vi "Bundle Script_Named (Un)Bundler Rearrange.vi"(8 "error in":errorcluster, 10 "Displayed Items":string[](array[string]), 11 "Affected Items":T1) -> (0 "error out":errorcluster, 2 "Objects":refnum<vi>[](array[refnum]))   [LabVIEW 2023]
doc: "Tag tree tags as nput, as these contain the original indices, which are used for reordering the wires and labels of the bundle or unbundle by name structures"
uses:
  top/BundleMagic.ctl
panel:
  out "Array":cluster{"Array":bool[]}[](array[cluster])
  out "Bundle Type":T2(ring)
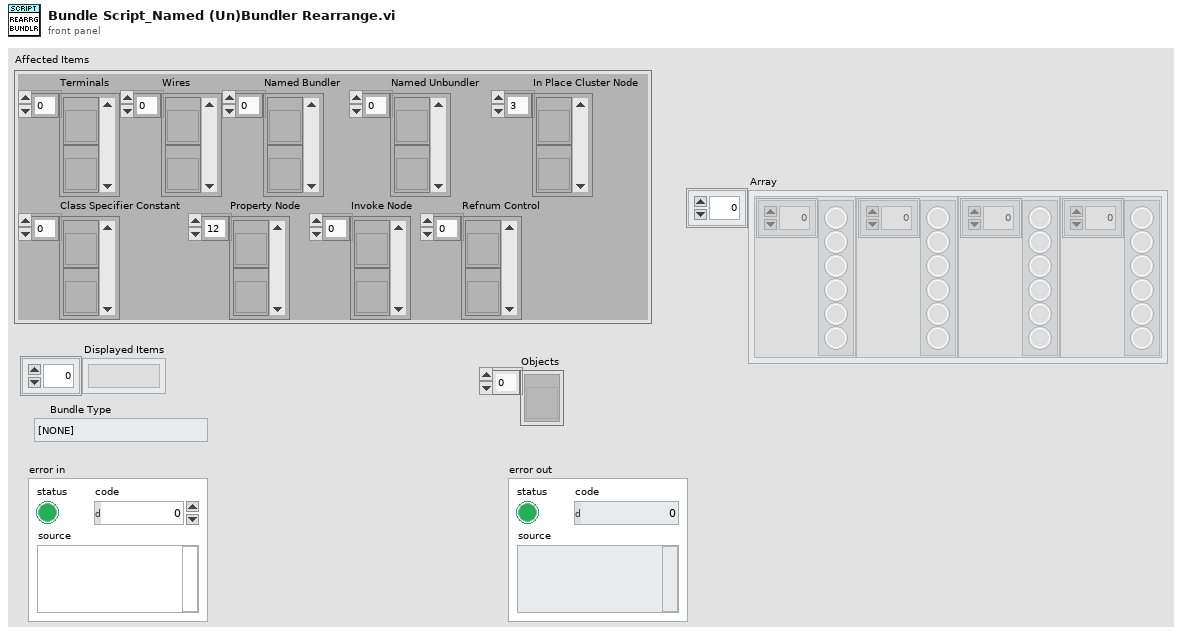
[diagram p1: front panel]
types:
  T1 = typedef "BundleMagic.ctl" = cluster{"Terminals":refnum<vi>[], "Wires":refnum<vi>[], "Named Bundler":refnum<vi>[], "Named Unbundler":refnum<vi>[], "In Place Cluster Node":refnum<vi>[], "Class Specifier Constant":refnum<vi>[], "Property Node":refnum<vi>[], "Invoke Node":refnum<vi>[], "Refnum Control":refnum<vi>[]}
  T2 = enum16{"[NONE]", "Unbundle", "Bundle", "Insert Before", "Insert After", "Remove Elements", "Rearrange Elements"}
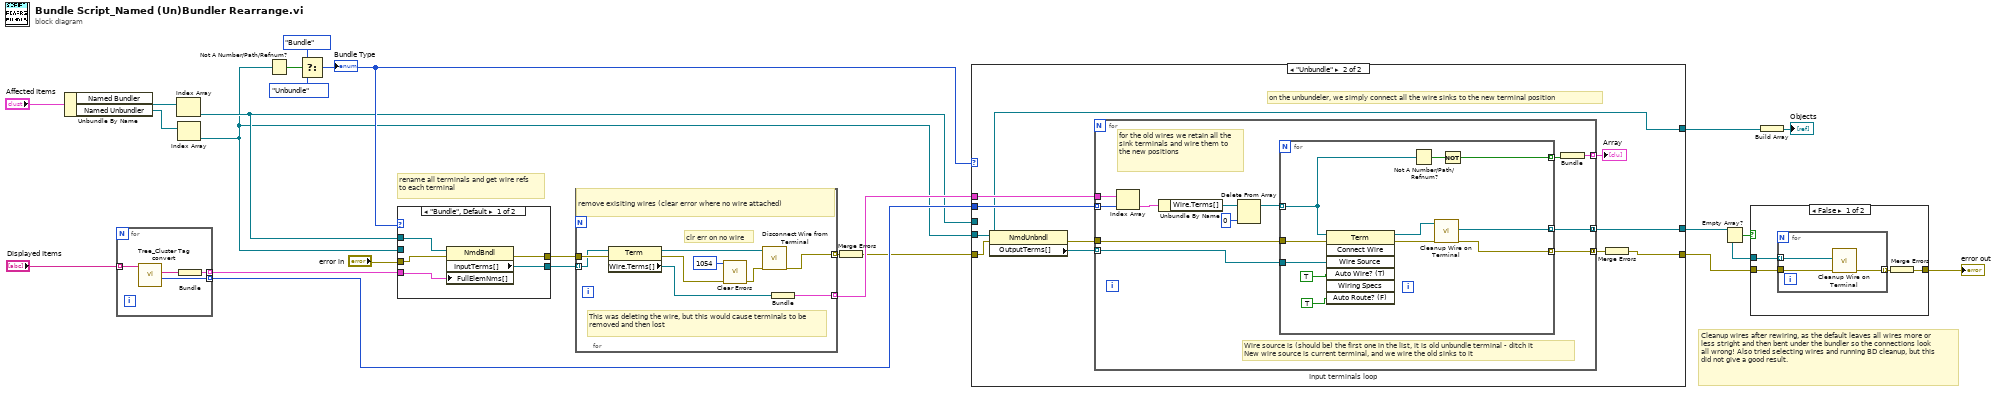
[diagram p0: block diagram]
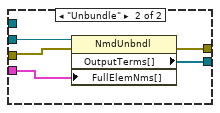
[diagram p2: hidden frame]
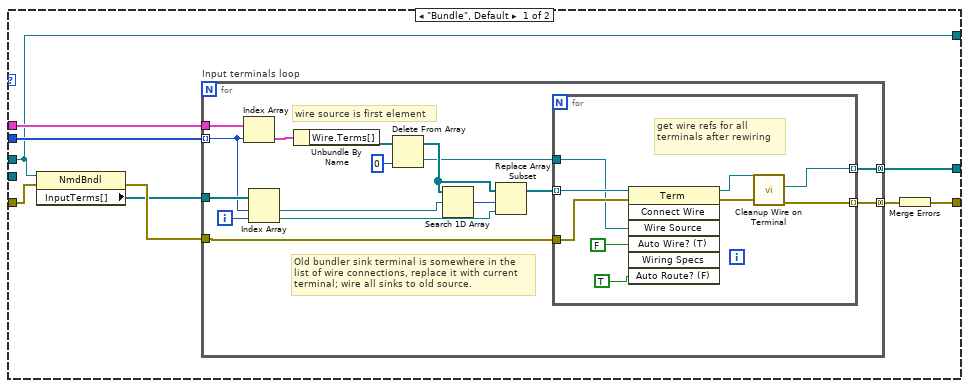
[diagram p3: hidden frame]
diagram:
  # "Cleanup wires after rewiring, as the default leaves all wires more or less stright and then bent under the bundler so the connections look all wrong! Also tried selecting wires and running BD cleanup, but this did not give a good result."
  # "rename all terminals and get wire refs to each terminal"
  n1 = Unbundle By Name("Affected Items") -> ("Named Bundler"=w14:refnum<vi>[], "Named Unbundler"=w12:refnum<vi>[])
  n2 = for {
    tunnel: "Displayed Items" -> [w28] mode=indexing
    tunnel: [w25] -> w17 mode=indexing
    tunnel: [w26] -> w19 mode=indexing
    n3 = call "Tree_Cluster Tag convert.vi"("Tag"=w28) -> ("Index"=w26:u32, "Tree Nest"=w27:string[])  [unwired: 5 in, 4 out]
    n4 = Bundle("Tree Nest"=w27) -> (w25:cluster{"Tree Nest":string[]})  [unwired: 1 in]
  }
  n5 = Index Array(array=w14) -> (element=w11:refnum<vi>)  [unwired: 1 in]
  n6 = Index Array(array=w12) -> (element=w9:refnum<vi>)  [unwired: 1 in]
  n7 = Not A Number/Path/Refnum?(number/path/refnum=w9) -> (NaN/Path/Refnum?=w10:bool)
  n8 = Select(t=T2."Bundle" ("Action"), s=w10, f=T2."Unbundle" ("Action")) -> (s? t:f=w16:T2)
  "Bundle Type" <- w16
  n9 = case shown="\"Bundle\", Default" w16 {
    tunnel: [w30 w38] -> w21
    tunnel: [w31 w37] -> w24
    tunnel: w11 -> [w33 _]
    tunnel: w17 -> [w32 w35]
    tunnel: w9 -> [_ w36]
    tunnel: "error in" -> [w29 w34]
    frame "Bundle", Default {
      n10 = property class="NmdBndl"(reference=w33, error in=w29, "FullElemNms[]"=w32) -> (error out=w31:errorcluster, "InputTerms[]"=w30:refnum<vi>[])  [unwired: 1 out]
    }
    frame "Unbundle" {
      n11 = property class="NmdUnbndl"(reference=w36, error in=w34, "FullElemNms[]"=w35) -> (error out=w37:errorcluster, "OutputTerms[]"=w38:refnum<vi>[])  [unwired: 1 out]
    }
  }
  n12 = for {
    tunnel: w21 -> [w46] mode=indexing
    tunnel: [w44] -> w20 mode=indexing
    tunnel: w24 -> [w47]
    tunnel: [w41] -> w18 mode=indexing
    # "This was deleting the wire, but this would cause terminals to be removed and then lost"
    # "clr err on no wire"
    # "remove exisiting wires (clear error where no wire attached)"
    n13 = property class="Term"(reference=w46, error in=w47) -> (reference out=w43:refnum<vi>, error out=w42:errorcluster, "Wire.Terms[]"=w45:refnum<vi>[])
    n14 = call <vilib>:"Clear Errors.vi"("error in (no error)"=w42, "specific error code to clear (0: all)"=1054) -> ("error out"=w40:errorcluster)  [unwired: 4 in, 1 out]
    n15 = call "Disconnect Wire from Terminal.vi"("error in"=w40, "Terminal in"=w43) -> ("error out"=w41:errorcluster)  [unwired: 5 in, 4 out]
    n16 = Bundle("Wire.Terms[]"=w45) -> (w44:cluster{"Wire.Terms[]":refnum<vi>[]})  [unwired: 1 in]
  }
  n17 = Merge Errors(w18) -> (w1:errorcluster)
  n18 = case shown="\"Unbundle\"" w16 {
    tunnel: w1 -> [w53 w88]
    tunnel: w20 -> [w55 w90]
    tunnel: w11 -> [w49 _]
    tunnel: w9 -> [_ w83]
    tunnel: w19 -> [w52 w87]
    tunnel: [w51 w85] -> w3
    tunnel: [w48 w82] -> w8
    tunnel: [w49 w83] -> w5
    frame "Bundle", Default {
      n19 = property class="NmdBndl"(reference=w49, error in=w53) -> (error out=w56:errorcluster, "InputTerms[]"=w54:refnum<vi>[])  [unwired: 1 out]
      n20 = for "Input terminals loop" {
        tunnel: w55 -> [w71]
        tunnel: w52 -> [w68] mode=indexing
        tunnel: w54 -> [w69]
        tunnel: w56 -> [w72]
        tunnel: [w58] -> w51 mode=concatenating
        tunnel: [w57] -> w50 mode=concatenating
        i -> [w67]
        # "wire source is first element"
        # "Old bundler sink terminal is somewhere in the list of wire connections, replace it with current terminal; wire all sinks to old source."
        n21 = Index Array(array=w71, index=w68) -> (element=w70:cluster{"Wire.Terms[]":refnum<vi>[]})
        n22 = Index Array(array=w69, index #1=w68, index #2=w67) -> (element #1=w65:refnum<vi>, element #2=w63:refnum<vi>)
        n23 = Unbundle By Name(w70) -> ("Wire.Terms[]"=w66:refnum<vi>[])
        n24 = Delete From Array(array=w66, index=0) -> (deleted portion=w59:refnum<vi>, array with subset deleted=w61:refnum<vi>[])  [unwired: 1 in]
        n25 = Search 1D Array(1D array=w61, element=w65) -> (index of element=w64:i32)  [unwired: 1 in]
        n26 = Replace Array Subset(array=w61, new element=w63, index=w64) -> (w62:refnum<vi>[])
        n27 = for {
          tunnel: w72 -> [w81]
          tunnel: w62 -> [w80] mode=indexing
          tunnel: w59 -> [w78]
          tunnel: [w74] -> w58 mode=indexing
          tunnel: [w73] -> w57 mode=indexing
          # "get wire refs for all terminals after rewiring"
          n28 = invoke class="Term" method="Connect Wire"(reference=w80, error in=w81, "Wire Source"=w78, "Auto Wire? (T)"=FALSE, "Auto Route? (F)"=TRUE) -> (reference out=w75:refnum<vi>, error out=w76:errorcluster)  [unwired: 2 in, 5 out]
          n29 = call "Cleanup Wire on Terminal.vi"("error in"=w76, "Terminal in"=w75) -> ("error out"=w73:errorcluster, "Wire out"=w74:refnum<vi>)  [unwired: 7 in, 1 out]
        }
      }
      n30 = Merge Errors(w50) -> (w48:errorcluster)
    }
    frame "Unbundle" {
      # "on the unbundeler, we simply connect all the wire sinks to the new terminal position"
      n31 = property class="NmdUnbndl"(reference=w83, error in=w88) -> (error out=w91:errorcluster, "OutputTerms[]"=w89:refnum<vi>[])  [unwired: 1 out]
      n32 = for "Input terminals loop" {
        tunnel: w90 -> [w100]
        tunnel: w87 -> [w98] mode=indexing
        tunnel: w91 -> [w103]
        tunnel: w89 -> [w101] mode=indexing
        tunnel: [w96] -> w85 mode=concatenating
        tunnel: [w95] -> w86 mode=concatenating
        tunnel: [w92] -> w84 mode=indexing
        # "for the old wires we retain all the sink terminals and wire them to the new positions"
        # "Wire source is (should be) the first one in the list, it is old unbundle terminal - ditch it\nNew wire source is current terminal, and we wire the old sinks to it"
        n33 = Index Array(array=w100, index=w98) -> (element=w99:cluster{"Wire.Terms[]":refnum<vi>[]})
        n34 = Unbundle By Name(w99) -> ("Wire.Terms[]"=w102:refnum<vi>[])
        n35 = Delete From Array(array=w102, index=0) -> (array with subset deleted=w94:refnum<vi>[])  [unwired: 1 in, 1 out]
        n36 = for {
          tunnel: w103 -> [w114]
          tunnel: w94 -> [w110] mode=indexing
          tunnel: w101 -> [w112]
          tunnel: [w107] -> w96 mode=indexing
          tunnel: [w105] -> w95 mode=indexing
          tunnel: [w108] -> w93 mode=indexing
          n37 = invoke class="Term" method="Connect Wire"(reference=w110, error in=w114, "Wire Source"=w112, "Auto Wire? (T)"=TRUE ("Auto Route? (F)"), "Auto Route? (F)"=TRUE) -> (reference out=w104:refnum<vi>, error out=w106:errorcluster)  [unwired: 2 in, 5 out]
          n38 = Not A Number/Path/Refnum?(number/path/refnum=w110) -> (NaN/Path/Refnum?=w109:bool)
          n39 = call "Cleanup Wire on Terminal.vi"("error in"=w106, "Terminal in"=w104) -> ("error out"=w105:errorcluster, "Wire out"=w107:refnum<vi>)  [unwired: 7 in, 1 out]
          n40 = Not(x=w109) -> (.not. x?=w108:bool)
        }
        n41 = Bundle(w93) -> (w92:cluster{bool[]})  [unwired: 1 in]
      }
      "Array" <- w84
      n42 = Merge Errors(w86) -> (w82:errorcluster)
    }
  }
  n43 = Empty Array?(array=w3) -> (empty?=w2:bool)
  n44 = case shown="False" w2 {
    tunnel: w3 -> [w118 _]
    tunnel: w8 -> [w117 w122]
    tunnel: [w115 w122] -> w7
    frame False {
      n45 = for {
        tunnel: w118 -> [w119] mode=indexing
        tunnel: w117 -> [w121]
        tunnel: [w120] -> w116 mode=indexing
        n46 = call "Cleanup Wire on Terminal.vi"("error in"=w121, "Wire In"=w119) -> ("error out"=w120:errorcluster)  [unwired: 7 in, 2 out]
      }
      n47 = Merge Errors(w116) -> (w115:errorcluster)
    }
    frame True {
    }
  }
  "error out" <- w7
  n48 = Build Array(w5) -> (→"Objects":refnum<vi>[])
